vi "OAT Even Time or Speed Segment (XY).vi"(0 "XY signal":cluster{"X":dbl[], "Y":dbl[]} {"X" format="%.2f"; "Y" format="%.2f"}, 1 "x-axis selection":u16(ring)=2 items=["Time", "Revolution", "RPM"], 2 "reset? (F)":bool, 3 "phase input? (F)":bool, 5 "speed profile":T4 {"speed [RPM]" format="%.2f"; "time [s]" format="%.2f"}, 7 "position info":T2, 9 "pulse/revolution (1)":i32=1, 11 "error in (no error)":errorcluster, 12 "segment settings":cluster{"start":dbl, "end":dbl, "step size":dbl} {"step size" format="%.2f"; "end" min=0.0 format="%.2f"; "start" min=0.0 format="%.2f"}, 13 "view info":T1={"dB on? (F)"=FALSE, "unwrap phase? (T)"=TRUE, "unit in degree? (T)"=TRUE}) -> (4 "XY signal out":cluster{"X":dbl[], "Y":dbl[]} {"X" format="%.2f"; "Y" format="%.2f"}, 8 "position info out":T2, 10 "end reached?":bool, 14 "actual segment settings":T3 {"actual step size" format="%.2f"; "actual end" min=0.0 format="%.2f"; "actual start" min=0.0 format="%.2f"}, 15 "error out":errorcluster)   [LabVIEW 2017, in "SoundVib_OAUtility.lvlib"]
doc: "Divides an input signal into even-time segments or even-speed intervals. The input signal of this VI can be an even-angle signal or an XY signal. When you use this VI to divide an XY signal, the XY signal can be only the output of the OAT Order Magnitude and Phase VI or OAT Overall Level Plot VI. Wire data to the <B>even-angle signal</B> input to determine the polymorphic instance to use or manually select the instance."
uses:
  <vilib>/addons/Sound and Vibration/Order Analysis/Utility/SoundVib_OAUtility.lvlib
  <vilib>/addons/Sound and Vibration/Order Analysis/Tach Process/SubVIs/speed profile.ctl
  <vilib>/addons/Sound and Vibration/Order Analysis/Misc/OAT Position Info.ctl
  <vilib>/addons/Sound and Vibration/Order Analysis/Tach Process/SoundVib_TachProcess.lvlib
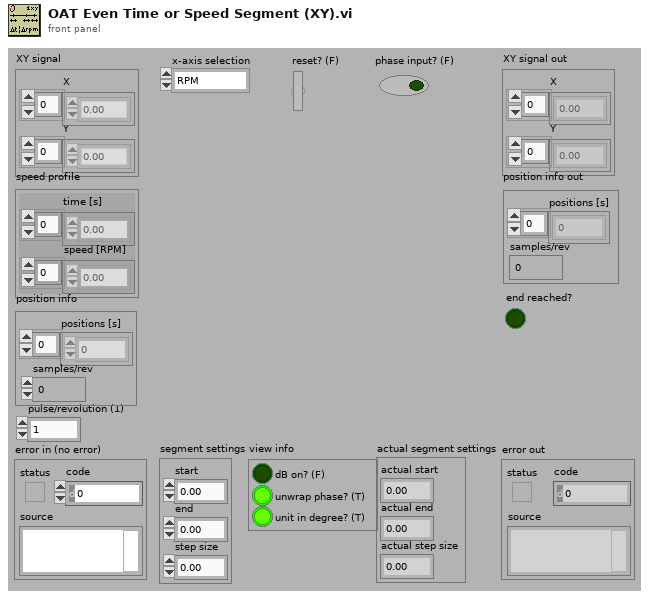
[diagram p1: front panel]
types:
  T1 = cluster{"dB on? (F)":bool, "unwrap phase? (T)":bool, "unit in degree? (T)":bool}
  T2 = typedef "OAT Position Info.ctl" = cluster{"positions [s]":dbl[], "samples/rev":dbl}
  T3 = cluster{"actual start":dbl, "actual end":dbl, "actual step size":dbl}
  T4 = typedef "SoundVib_TachProcess.lvlib/speed profile.ctl" = cluster{"time [s]":dbl[], "speed [RPM]":dbl[]}
  T5 = cluster{"last rev":dbl, "rev indice":dbl[], "time indice":dbl[], "RPM indice":dbl[]}
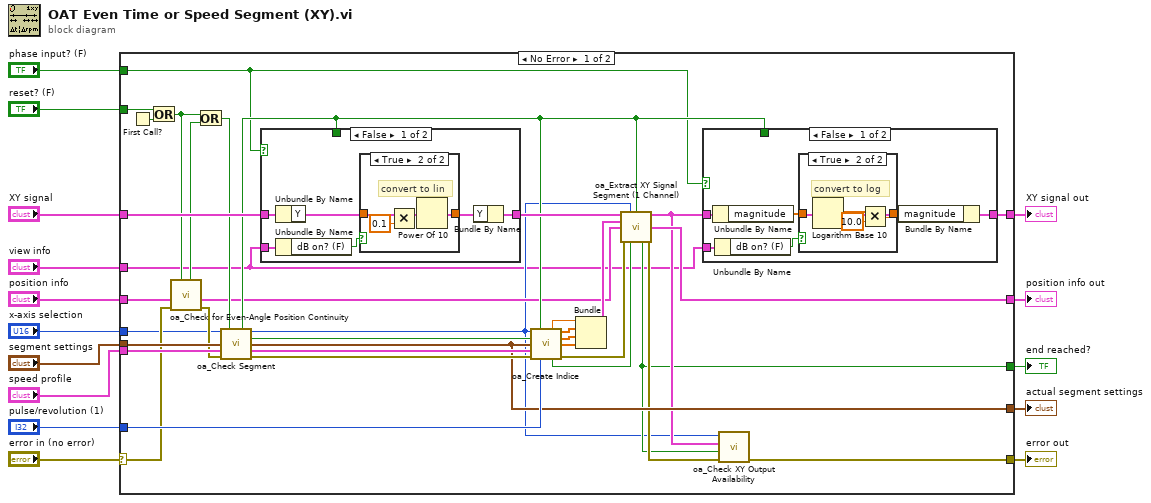
[diagram p0: block diagram]
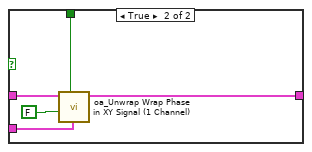
[diagram p3: hidden frame]
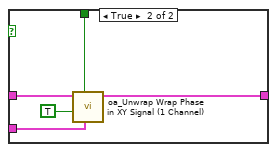
[diagram p5: hidden frame]
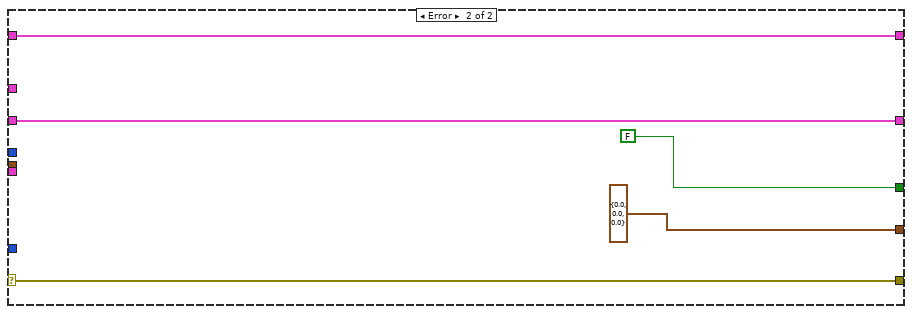
[diagram p6: hidden frame]
diagram:
  n1 = case shown="No Error" "error in (no error)" {
    selector: "error in (no error)" -> [w25 w88]
    tunnel: [w22 w88] -> w14
    tunnel: "reset? (F)" -> [w34 _]
    tunnel: "x-axis selection" -> [w19 _]
    tunnel: "segment settings" -> [w44 _]
    tunnel: "speed profile" -> [w29 _]
    tunnel: [w42 cluster{"start":dbl, "end":dbl, "step":dbl} {"start"=0.0, "end"=0.0, "step"=0.0} ("steps output")] -> w9
    tunnel: "pulse/revolution (1)" -> [w43 _]
    tunnel: "XY signal" -> [w37 w86]
    tunnel: [w20 FALSE ("finish?")] -> w6
    tunnel: "position info" -> [w40 w85]
    tunnel: [w35 w86] -> w4
    tunnel: [w38 w85] -> w3
    tunnel: "phase input? (F)" -> [w17 _]
    tunnel: "view info" -> [w16 _]
    frame No Error {
      n2 = First Call?() -> (First Call?: T/F=w33:bool)
      n3 = Or(x=w34, y=w33) -> (x .or. y?=w27:bool)
      n4 = call <vilib>:"oa_Check for Even-Angle Position Continuity.vi"("reset in"=w27, "error in (no error)"=w25, "even-angle position info"=w40) -> ("error out"=w24:errorcluster, "even-angle position info dup"=w28:T2, "position not continuous"=w26:bool)  [unwired: 6 in]
      n5 = Or(x=w27, y=w26) -> (x .or. y?=w30:bool)
      n6 = call <vilib>:"oa_Check Segment.vi"("X axis selection"=w19, "reset?(F)"=w30, "segment position"=w44, "speed profile"=w29, "error in (no error)"=w24) -> ("reset out"=w31:bool, "X axis selection"=w18:u16, "step found?"=w49:bool, "segment position out"=w42:cluster{"start":dbl, "end":dbl, "step size":dbl}, "dul speed profile"=w50:T4, "error out"=w51:errorcluster)  [unwired: 5 in]
      n7 = case shown="False" w17 {
        tunnel: w37 -> [w73 w83]
        tunnel: [w72 w82] -> w36
        tunnel: w16 -> [w71 w79]
        tunnel: w31 -> [_ w81]
        frame False {
          n8 = Unbundle By Name(w73) -> ("Y"=w69:dbl[])
          n9 = Unbundle By Name(w71) -> ("dB on? (F)"=w70:bool)
          n10 = case shown="True" w70 {
            tunnel: w69 -> [w74 w77]
            tunnel: [w74 w78] -> w68
            frame False {
            }
            frame True {
              # "convert to lin"
              n11 = Multiply(x=w77, y=0.1) -> (x*y=w76:dbl[])
              n12 = Power Of 10(x=w76) -> (10^x=w78:dbl[])
            }
          }
          n13 = Bundle By Name(cluster=w73, "Y"=w68) -> (w72:cluster{"X":dbl[], "Y":dbl[]})
        }
        frame True {
          n14 = call <vilib>:"oa_Unwrap Wrap Phase in XY Signal (1 Channel).vi"("view"=w79, "reset? (F)"=w81, "Unwrap?"=TRUE, "XY signal"=w83) -> ("XY signal out"=w82:cluster{"X":dbl[], "Y":dbl[]})  [unwired: 7 in]
        }
      }
      n15 = call <vilib>:"oa_Create Indice.vi"("X axis selection"=w18, "reset?(F)"=w31, "step found?(F)"=w49, "steps input"=w42, "speed profile"=w50, "error in (no error)"=w51, "pulse/revolution (1)"=w43) -> ("last rev"=w45:dbl, "rev indice"=w46:dbl[], "time indice"=w47:dbl[], "RPM indice"=w48:dbl[], "reach end?"=w32:bool, "error out"=w39:errorcluster)  [unwired: 2 in, 1 out]
      n16 = Bundle("last rev"=w45, "rev indice"=w46, "time indice"=w47, "RPM indice"=w48) -> (w41:T5)  [unwired: 1 in]
      n17 = call <vilib>:"oa_Extract XY Signal Segment (1 Channel).vi"("XY signal in"=w36, "X axis selection"=w18, "reset? (F)"=w31, "trigger indices"=w41, "position info in"=w28, "error in (no error)"=w39, "indices end?"=w32) -> ("XY signal out"=w21:cluster{"time/rev/rpm":dbl[], "magnitude":dbl[]}, "position info out"=w38:T2, "reached end?"=w20:bool, "error out"=w23:errorcluster)  [unwired: 5 in]
      n18 = case shown="False" w17 {
        tunnel: w21 -> [w53 w67]
        tunnel: [w52 w66] -> w35
        tunnel: w31 -> [_ w64]
        tunnel: w16 -> [w57 w63]
        frame False {
          n19 = Unbundle By Name(w53) -> ("magnitude"=w55:dbl[])
          n20 = Unbundle By Name(w57) -> ("dB on? (F)"=w54:bool)
          n21 = case shown="True" w54 {
            tunnel: w55 -> [w58 w62]
            tunnel: [w58 w61] -> w56
            frame False {
            }
            frame True {
              # "convert to log"
              n22 = Logarithm Base 10(1:w62) -> (0:w59:dbl[])
              n23 = Multiply(x=w59, y=10.0) -> (x*y=w61:dbl[])
            }
          }
          n24 = Bundle By Name(cluster=w53, "magnitude"=w56) -> (w52:cluster{"time/rev/rpm":dbl[], "magnitude":dbl[]})
        }
        frame True {
          n25 = call <vilib>:"oa_Unwrap Wrap Phase in XY Signal (1 Channel).vi"("view"=w63, "reset? (F)"=w64, "Unwrap?"=FALSE, "XY signal"=w67) -> ("XY signal out"=w66:cluster{"X":dbl[], "Y":dbl[]})  [unwired: 7 in]
        }
      }
      n26 = call <vilib>:"oa_Check XY Output Availability.vi"("error in (no error)"=w23, "reached end?"=w20, "XY signal"=w21, "x-axis selection"=w18) -> ("error out"=w22:errorcluster)  [unwired: 7 in]
    }
    frame Error {
    }
  }
  "error out" <- w14
  "XY signal out" <- w4
  "end reached?" <- w6
  "actual segment settings" <- w9
  "position info out" <- w3
